vi "Configure Connection Collection.vi"(5 "Connection":refnum<class "Connection.Collection.lvclass">, 6 "timeout (-1: Connection Default)":i32=5000, 8 "error in (no error)":errorcluster, 11 "Collection":refnum<class "Connection.lvclass">[](array[class])) -> (0 "error out":errorcluster, 3 "Connection":refnum<class "Connection.Collection.lvclass">)   [LabVIEW 2013, in "Connection_GOSPL.lvlib" / "Connection.Collection.lvclass"]
uses:
  Connection.Collection.lvclass
  Connection/Connection.lvclass
  Connection/Connection.lvclass/Connection.ctl
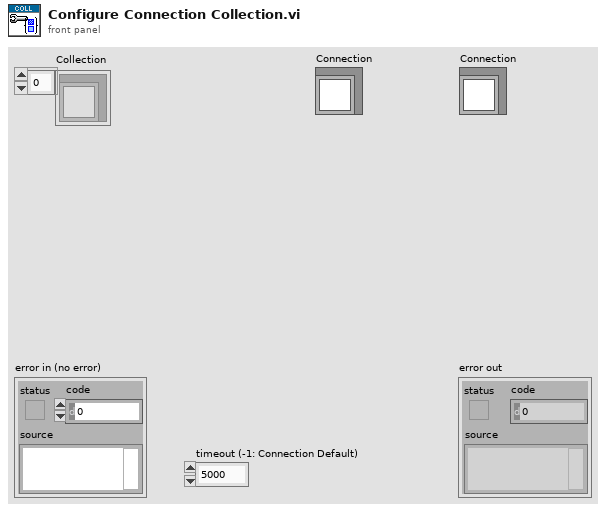
[diagram p1: front panel]
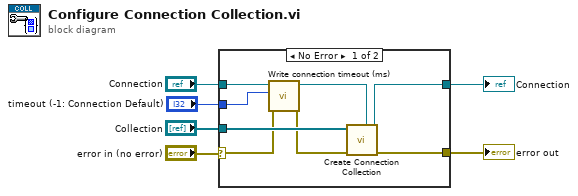
[diagram p0: block diagram]
diagram:
  n1 = case shown="No Error" "error in (no error)" {
    selector: "error in (no error)" -> [w8 w16]
    tunnel: [w12 w16] -> w5
    tunnel: [w13 w15] -> w3
    tunnel: "Collection" -> [w14 _]
    tunnel: "Connection" -> [w10 w15]
    tunnel: "timeout (-1: Connection Default)" -> [w11 _]
    frame No Error {
      n2 = call "Write connection timeout (ms).vi"("error in (no error)"=w8, "connection timeout (ms)"=w11, "Connection in"=w10) -> ("error out"=w7:errorcluster, "Connection out"=w9:refnum<class "Connection.Collection.lvclass">)  [unwired: 7 in]
      n3 = call "Create Connection Collection.vi"("Connection.Collection"=w9, "error in (no error)"=w7, "Collection"=w14) -> ("error out"=w12:errorcluster, "Connection.Collection"=w13:refnum<class "Connection.Collection.lvclass">)  [unwired: 7 in]
    }
    frame Error {
    }
  }
  "error out" <- w5
  "Connection" <- w3
